vi "Initialise_3D_Mesh.vi"(8 "Gain":dbl[](array[numeric]), 9 "Size":i32[](array[numeric])=[-116, 4240, 19456, 581, 494, 15616, -1831, 531, 16640, -1384, 2689, 18688, -3717, 1780, 17664, 103, 6163, 16384, -435, -1091, 16384, 6061, 5490, 17664, 994, 6404, 17408, 7175, 2119, 15616, 6696, 4445, 13056, 3779, 4292, 15360, 6211, 2706, 13312, -879, 694, 18176, 1825, -926, 13824, 25, 522, 19968, 2701, -2574, 18688, 820, 2301, 18176, 8209, 355, 15616, 7530, 3049, 15872, 9036, 47, 14848, 8160, 1730, 15104, 8670, 3492, 14592, 6673, -707, 16384, 3422, 3530, 17408, -1725, 2172, 17664, 3006, 216, 14592, -3610, 78, 17408, -3524, -1404, 15616, -3464, 3718, 14848, -731, 310, -24576, -5419, -1055, 14592, 62, 684, 18688, 3029, -1500, 14592, -4748, -2744, 15104, 4310, -986, 14848, 1880, -1396, 16384, 1655, -408, 16640, 6378, 1963, 16384, 6643, 59, 13824, 6410, 1507, 19712, 3234, -1034, 14592, 2074, -2596, 16128, 2317, -3056, 17920, 1190, -2711, 14336, 1830, -5779, 17920, -2321, -3878, 16640, -1656, -5739, 17152, 4615, 144, 14848, 5972, 1941, 16128, 5218, 925, 13568, 8043, 210, 16896, 8297, -1060, 14080, 6183, -10282, 13568, 3113, -695, 17664, -1849, 82, 19712, 7031, -1846, 20224, 4588, -4442, 16384, 7182, -7779, 18688, 1244, -7134, -21504, 907, 6738, -23296, 3002, -80, 16640, 4025, -3886, 16384, 4135, -6244, 18688], 10 "Y Coords":dbl[](array[numeric]), 11 "X Coords":dbl[](array[numeric])) -> (3 "SceneMesh out":refnum<vi>, 5 "3D Plot Data":T1)   [LabVIEW 2016]
uses:
  controls/3D_Plot_Data.ctl
  <vilib>/picture/3D Picture Control/NI_3D Picture Control.lvlib
panel:
  out "Init Vertex Array":cluster{"x":dbl, "y":dbl, "z":dbl}[](array[cluster])
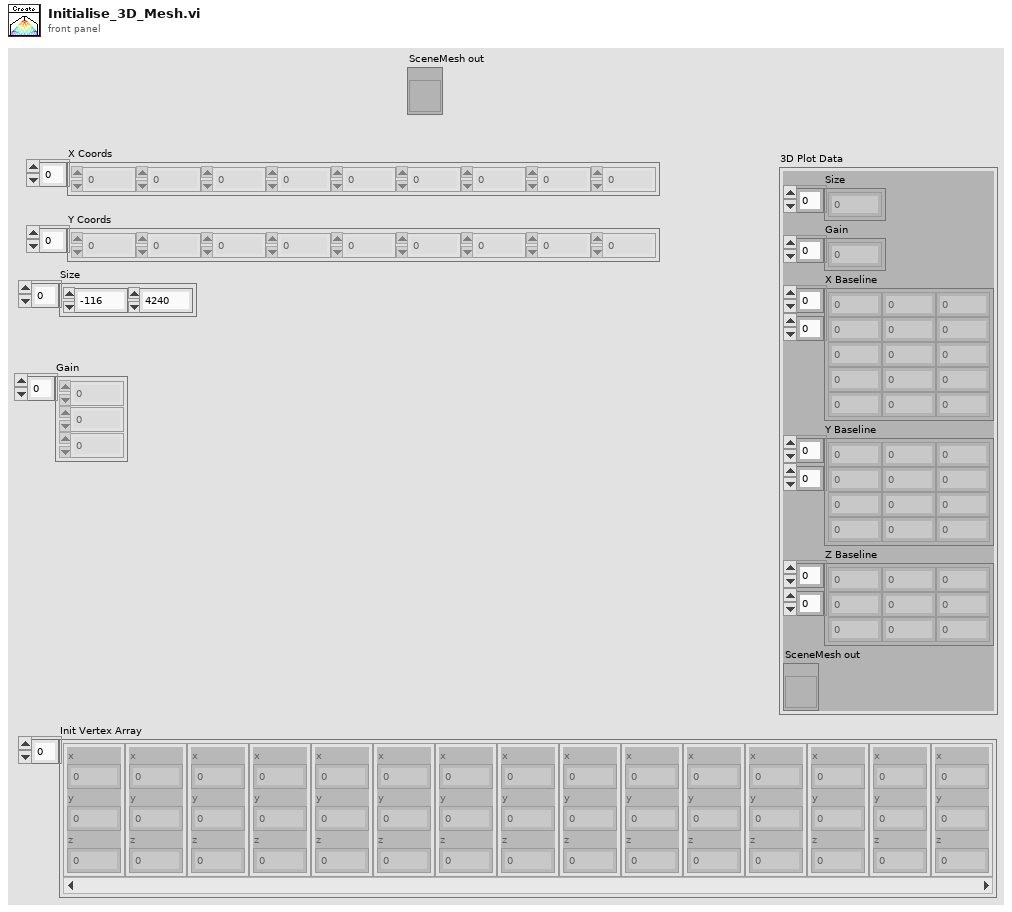
[diagram p1: front panel]
types:
  T1 = typedef "3D_Plot_Data.ctl" = cluster{"Size":i32[], "Gain":dbl[], "X Baseline":dbl[][], "Y Baseline":dbl[][], "Z Baseline":dbl[][], "SceneMesh out":refnum<vi>}
  T2 = cluster{"Red":sgl, "Green":sgl, "Blue":sgl, "Alpha":sgl}[]
  T3 = enum16{"Overall", "Per Primitive", "Per Vertex", "Binding Off"}
  T4 = enum16{"Points", "Lines", "Line Strip", "Line Loop", "Triangles", "Triangle Strip", "Triangle Fan", "Quads", "Quad Strip", "Polygon"}
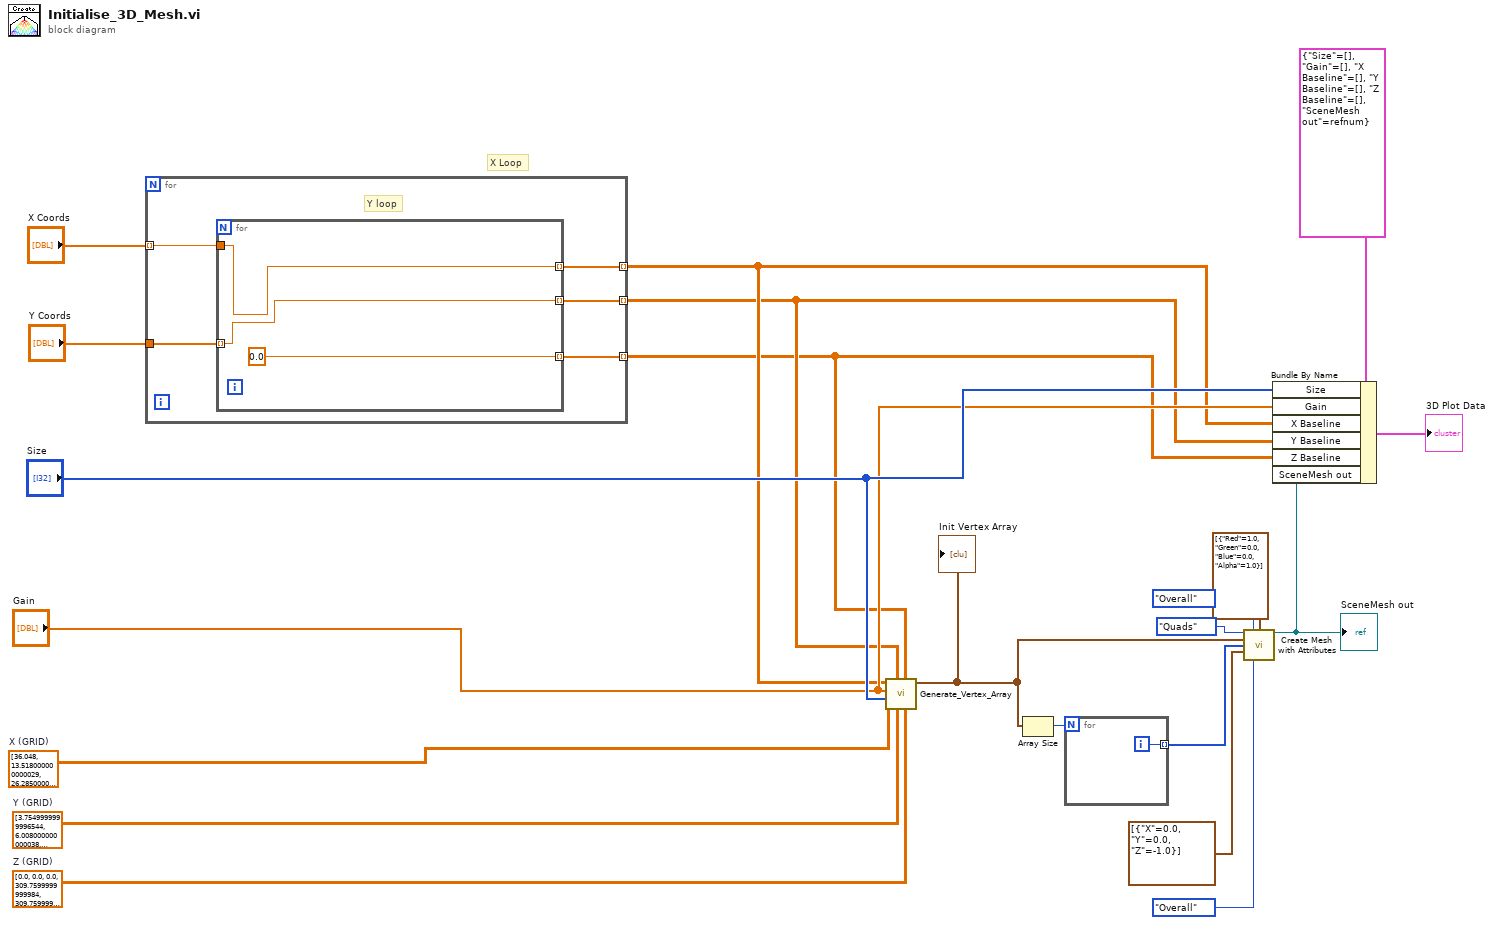
[diagram p0: block diagram]
diagram:
  w10 = dbl[][] [[36.048, 13.518000000000029, 26.285000000000082, 40.55400000000009, 22.529999999999745, 39.803, 24.783000000000015, 12.766999999999825], [27.035999999999998, 57.07600000000002, -16.522000000000048, 171.97900000000027, 122.41300000000001, 135.93099999999959, 114.90300000000025, 21.778999999999996], [14.269000000000005, 3.7549999999999955, 817.0879999999997, 467.1219999999994, 445.34299999999985, 379.2550000000001, 228.3040000000001, 99.1319999999996], [-2.2529999999997017, -50.31700000000001, -25.533999999999992, -117.15599999999995, -596.2940000000003, 227.55299999999988, -26.284999999999854, 83.36099999999988], [-9.012, 25.534000000000106, -40.55400000000009, 115.654, -18.023999999999887, 5.257000000000062, 208.77799999999934, 147.1959999999999], [-23.28099999999995, -17.27299999999991, 13.518000000000029, 10.51400000000001, 28.53800000000001, 22.529999999999973, 57.82699999999977, 97.63000000000011], [-18.023999999999887, -29.289000000000215, -12.015999999999622, 0.0, 15.019999999999527, 34.54599999999982, 45.05999999999949, 29.28899999999976], [-21.027999999999793, -24.031999999999698, -24.7829999999999, 13.518000000000029, 11.264999999999986, 18.023999999999432, 6.008000000000266, -0.7510000000002037]]  # X (GRID)
  w9 = dbl[][] [[3.7549999999996544, 6.008000000000038, 12.766999999999996, 30.791000000000167, 18.023999999999887, 0.0, -15.770999999999958, -13.518000000000029], [10.51400000000001, -9.763000000000034, 47.31299999999993, 85.6139999999998, 93.1239999999998, 52.570000000000164, 12.766999999999825, -12.015999999999622], [22.529999999999973, 60.07999999999993, 46.56200000000001, 295.894, -3.7550000000000026, -18.77500000000009, 36.79899999999998, -67.58999999999997], [6.008000000000038, 23.28099999999995, 44.309, -155.457, 31.542, -218.541, 25.534000000000106, 5.257000000000062], [2.252999999999986, -3.0039999999999054, -74.34900000000016, 3.7549999999999955, -9.76299999999992, -72.84700000000001, 17.27299999999991, -82.61], [19.52600000000075, -1.5019999999999527, -72.84700000000066, -46.5619999999999, -83.36099999999988, -90.11999999999989, -46.56200000000001, -46.5619999999999], [11.265, -4.5060000000000855, -40.55400000000009, -6.0079999999999245, 7.510000000000019, 6.0079999999999245, 9.011999999999944, -18.024], [-0.7509999999992942, 13.518000000000029, -2.253, 6.00800000000072, 0.7510000000002037, -11.265000000000327, -18.77500000000009, -8.260999999999967]]  # Y (GRID)
  w11 = dbl[][] [[0.0, 0.0, 0.0, 309.7599999999984, 309.7599999999984, 0.0, 0.0, 0.0], [0.0, 309.76000000000204, 619.5200000000004, 309.7600000000002, 619.5200000000004, 309.7600000000002, 0.0, 309.76000000000204], [0.0, 619.5200000000004, 2787.84, 1548.7999999999993, 929.2799999999988, 929.2800000000025, 309.76000000000204, 309.7599999999984], [0.0, 309.7599999999984, 1239.0400000000009, 2478.0800000000017, 3097.600000000002, 1548.7999999999993, 929.2799999999988, 619.5200000000004], [0.0, 0.0, 619.5200000000004, 929.2799999999988, 1239.0400000000009, 1239.0399999999972, 929.2799999999988, 309.76000000000204], [0.0, 0.0, 309.76000000000204, 309.7599999999984, 619.5200000000004, 619.5200000000004, 309.76000000000204, 309.76000000000204], [0.0, 0.0, 0.0, 0.0, 0.0, 0.0, 309.76000000000204, 309.7599999999984], [0.0, 0.0, 0.0, 0.0, 0.0, 0.0, 309.7599999999984, 0.0]]  # Z (GRID)
  # "X Loop"
  n1 = for {
    tunnel: "X Coords" -> [w26] mode=indexing
    tunnel: "Y Coords" -> [w25]
    tunnel: [w24] -> w5 mode=indexing
    tunnel: [w23] -> w3 mode=indexing
    tunnel: [w22] -> w4 mode=indexing
    # "Y loop"
    n2 = for {
      tunnel: w26 -> [w29]
      tunnel: w25 -> [w27] mode=indexing
      tunnel: [w29] -> w24 mode=indexing
      tunnel: [0.0 ("element")] -> w23 mode=indexing
      tunnel: [w27] -> w22 mode=indexing
    }
  }
  n3 = call "Generate_Vertex_Array.vi"("Sensor Z"=w11, "Z Baseline"=w3, "Sensor Y"=w9, "Y Baseline"=w4, "Sensor X"=w10, "Size"="Size", "Gain"="Gain", "X Baseline"=w5) -> ("Init Vertex Array"=w15:cluster{"x":dbl, "y":dbl, "z":dbl}[])  [unwired: 3 in]
  "Init Vertex Array" <- w15
  n4 = Array Size(array=w15) -> (size(s)=w16:i32)
  n5 = for {
    N: w16 -> [_]
    tunnel: [w30] -> w14 mode=indexing
    i -> [w30]
  }
  n6 = call <vilib>:"Create Mesh with Attributes.vi"("Draw Mode"=T4."Quads", "Color Binding Mode"=T3."Overall", "Color Array"=T2 [{"Red"=1.0, "Green"=0.0, "Blue"=0.0, "Alpha"=1.0}], "Vertex Array"=w15, "Indices"=w14, "Normal Array"=cluster{"X":sgl, "Y":sgl, "Z":sgl}[] [{"X"=0.0, "Y"=0.0, "Z"=-1.0}], "Normal Binding Mode"=T3."Overall") -> ("New Mesh Refnum"=w1:refnum<vi>)  [unwired: 7 in, 1 out]
  "SceneMesh out" <- w1
  n7 = Bundle By Name(cluster=T1 {"Size"=[], "Gain"=[], "X Baseline"=[], "Y Baseline"=[], "Z Baseline"=[], "SceneMesh out"=refnum} ("3D Plot Data"), "Size"="Size", "Gain"="Gain", "X Baseline"=w5, "Y Baseline"=w4, "Z Baseline"=w3, "SceneMesh out"=w1) -> (→"3D Plot Data":T1)
